vi "GetTime.vi"(7 "State":enum16{"Get Time", "Calculate Differential"}(ring), 8 "Total Seconds":string, 9 "Stored Seconds":string, 10 "Stored Minutes":string, 11 "Stored Hours":string) -> (0 "Elapsed Seconds":i32, 1 "Seconds":string, 2 "Minutes":string, 3 "Hours":string, 4 "Total Seconds Out":string, 5 "Total Elapsed Time":i32)   [LabVIEW 2017]
panel:
  out "Stored Minutes":i32
  out "Stored Hours":i32
  out "Stored Seconds":i32
  out "Current Seconds":i32
  out "Current Hours":i32
  out "Current Minutes":i32
  out "Seconds":string
  out "Hours":string
  out "Minutes":string
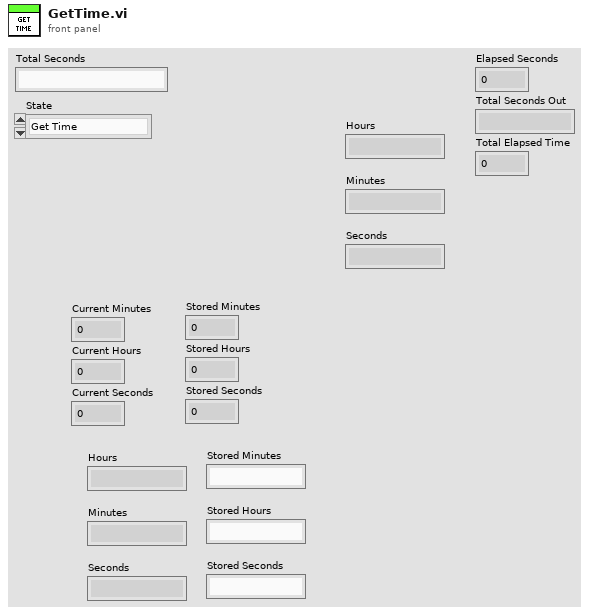
[diagram p1: front panel]
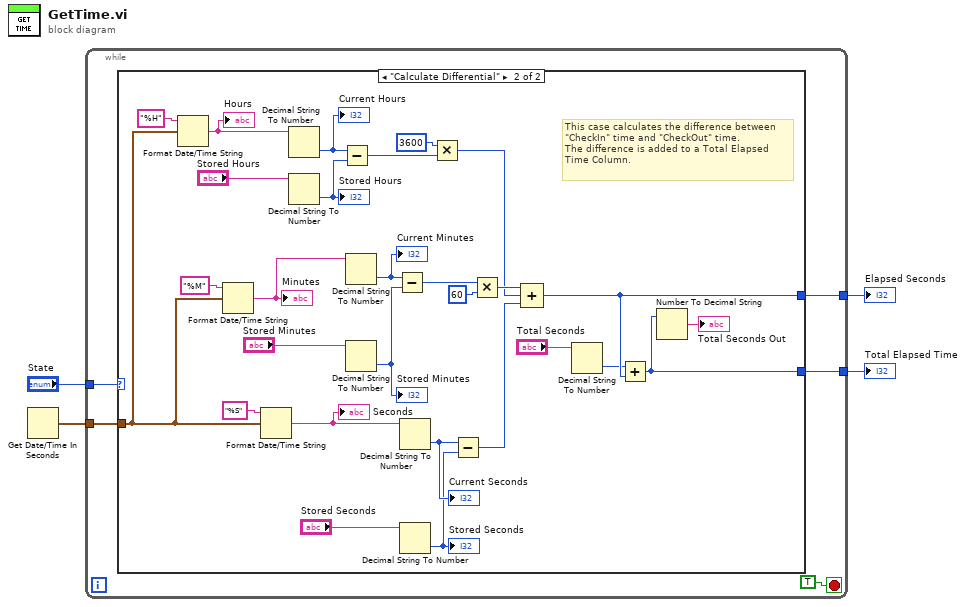
[diagram p0: block diagram]
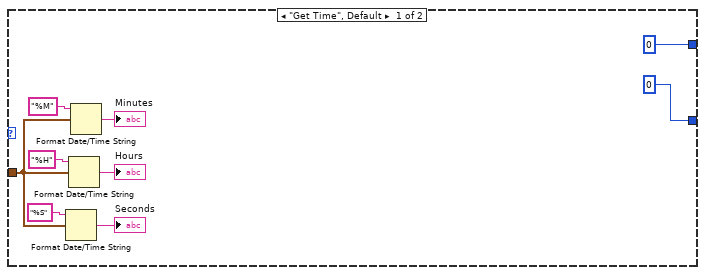
[diagram p2: hidden frame]
diagram:
  n1 = Get Date/Time In Seconds() -> (seconds since 1Jan1904=w4:timestamp)
  n2 = while {
    tunnel: w4 -> [w9]
    tunnel: "State" -> [w7]
    tunnel: [w6] -> w2
    tunnel: [w5] -> w1
    stop <- TRUE stop-if-true
    n3 = case shown="\"Calculate Differential\"" w7 {
      tunnel: w9 -> [w15 w43]
      tunnel: [0 w22] -> w6
      tunnel: [0 w19] -> w5
      frame "Get Time", Default {
        n4 = Format Date/Time String(time format string (%c)="%S", seconds (now)=w15) -> (date/time string=→"Seconds":string)  [unwired: 1 in]
        n5 = Format Date/Time String(time format string (%c)="%H", seconds (now)=w15) -> (date/time string=→"Hours":string)  [unwired: 1 in]
        n6 = Format Date/Time String(time format string (%c)="%M", seconds (now)=w15) -> (date/time string=→"Minutes":string)  [unwired: 1 in]
      }
      frame "Calculate Differential" {
        # "This case calculates the difference between\n\"CheckIn\" time and \"CheckOut\" time. \nThe difference is added to a Total Elapsed\nTime Column."
        n7 = Format Date/Time String(time format string (%c)="%H", seconds (now)=w43) -> (date/time string=w42:string)  [unwired: 1 in]
        "Hours" <- w42
        n8 = Format Date/Time String(time format string (%c)="%M", seconds (now)=w43) -> (date/time string=w41:string)  [unwired: 1 in]
        "Minutes" <- w41
        n9 = Format Date/Time String(time format string (%c)="%S", seconds (now)=w43) -> (date/time string=w40:string)  [unwired: 1 in]
        "Seconds" <- w40
        n10 = Decimal String To Number(string=w42) -> (number=w34:i32)  [unwired: 2 in, 1 out]
        "Current Hours" <- w34
        n11 = Decimal String To Number(string="Stored Hours") -> (number=w33:i32)  [unwired: 2 in, 1 out]
        "Stored Hours" <- w33
        n12 = Subtract(x=w34, y=w33) -> (x-y=w28:i32)
        n13 = Decimal String To Number(string=w41) -> (number=w36:i32)  [unwired: 2 in, 1 out]
        "Current Minutes" <- w36
        n14 = Decimal String To Number(string="Stored Minutes") -> (number=w35:i32)  [unwired: 2 in, 1 out]
        "Stored Minutes" <- w35
        n15 = Subtract(x=w36, y=w35) -> (x-y=w30:i32)
        n16 = Decimal String To Number(string=w40) -> (number=w32:i32)  [unwired: 2 in, 1 out]
        "Current Seconds" <- w32
        n17 = Decimal String To Number(string="Stored Seconds") -> (number=w31:i32)  [unwired: 2 in, 1 out]
        "Stored Seconds" <- w31
        n18 = Multiply(x=3600, y=w28) -> (x*y=w25:i32)
        n19 = Subtract(x=w32, y=w31) -> (x-y=w24:i32)
        n20 = Multiply(x=w30, y=60) -> (x*y=w26:i32)
        n21 = Compound Arithmetic op=ADD(w26, w25, w24) -> (w22:i32)
        n22 = Decimal String To Number(string="Total Seconds") -> (number=w21:i32)  [unwired: 2 in, 1 out]
        n23 = Add(x=w21, y=w22) -> (x+y=w19:i32)
        n24 = Number To Decimal String(number=w19) -> (decimal integer string=→"Total Seconds Out":string)  [unwired: 1 in]
      }
    }
  }
  "Elapsed Seconds" <- w2
  "Total Elapsed Time" <- w1
